vi "Read Thermometer with Save Path.vi"() -> ()   [LabVIEW 2020]
panel:
  in  "Path":path
  out "Waveform Chart":dbl(graph)
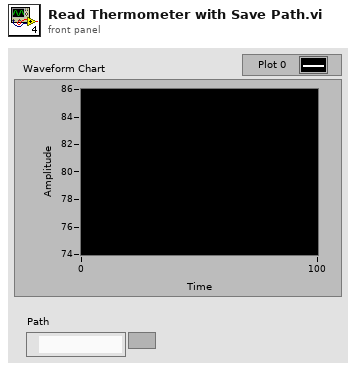
[diagram p1: front panel]
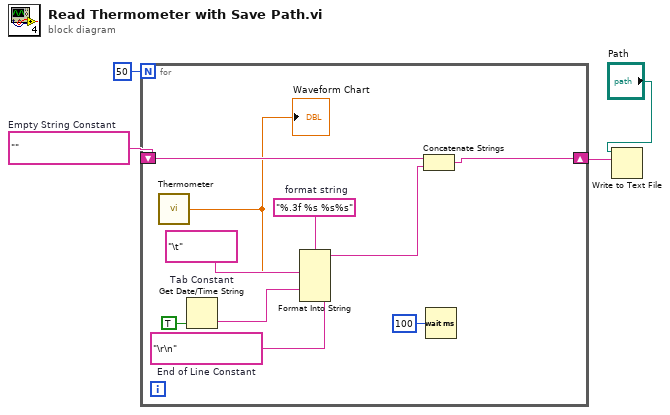
[diagram p0: block diagram]
diagram:
  w3 = ""  # Empty String Constant
  n1 = for {
    N: 50 -> [_]
    shift-right: [w8] -> w2
    shift-left: w3 -> [w10]
    w11 = "\r\n"  # End of Line Constant
    w7 = "\t"  # Tab Constant
    w14 = "%.3f %s %s%s"  # format string
    n2 = call "Thermometer.vi"() -> ("Temperature (deg F)"=w6:dbl)  [unwired: 1 in]
    "Waveform Chart" <- w6
    n3 = Get Date/Time String(want seconds? (F)=TRUE) -> (time string=w12:string)  [unwired: 2 in, 1 out]
    n4 = Format Into String "Format Into String"(format string=w14, w6, w7, w12, w11) -> (resulting string=w9:string)  [unwired: 2 in, 1 out]
    n5 = Concatenate Strings "Concatenate Strings"(w10, w9) -> (w8:string)
    n6 = Wait (ms)(milliseconds to wait=u32 100) -> ()  [unwired: 1 out]
  }
  n7 = Write to Text File(file (use dialog)="Path", text=w2) -> ()  [unwired: 2 in, 3 out]
